vi "text_message_to_gemini_message.vi"(2 "error in (no error)":errorcluster, 3 "message":T2) -> (0 "error out":errorcluster, 1 "Content (JSON)":string)   [LabVIEW 2020, in "llm_gemini_chatmodels.lvclass"]
uses:
  llm_gemini_chatmodels.lvclass
  message_text/message.ctl
  message_text/message_text.lvclass
panel:
  out "Content":T1
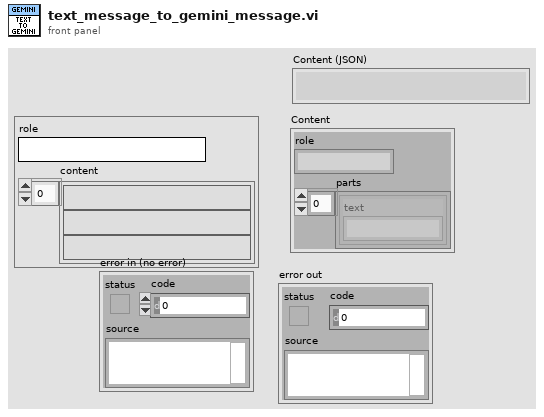
[diagram p1: front panel]
types:
  T1 = cluster{"role":string, "parts":cluster{"text":string}[]}
  T2 = typedef "message_text.lvclass/message.ctl" = cluster{"role":string, "content":string[]}
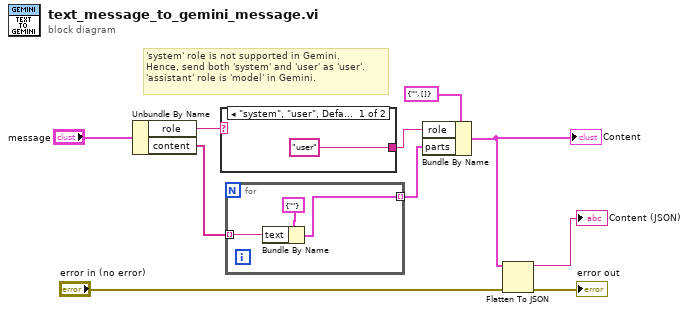
[diagram p0: block diagram]
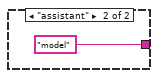
[diagram p2: hidden frame]
diagram:
  # "'system' role is not supported in Gemini.\nHence, send both 'system' and 'user' as 'user'.\n'assistant' role is 'model' in Gemini."
  n1 = Unbundle By Name("message") -> ("role"=w9:string, "content"=w6:string[])
  n2 = case shown="\"system\", \"user\", Default" w9 {
    tunnel: ["user" ("role") "model" ("role")] -> w8
    frame "system", "user", Default {
    }
    frame "assistant" {
    }
  }
  n3 = for {
    tunnel: w6 -> [w15] mode=indexing
    tunnel: [w13] -> w7 mode=indexing
    n4 = Bundle By Name(cluster=cluster{"text":string} {"text"=""} ("parts"), "text"=w15) -> (w13:cluster{"text":string})
  }
  n5 = Bundle By Name(cluster=T1 {"role"="", "parts"=[]} ("content"), "role"=w8, "parts"=w7) -> (w5:T1)
  "Content" <- w5
  n6 = Flatten To JSON(anything=w5, error in (no error)="error in (no error)") -> (JSON string=→"Content (JSON)":string, 11:→"error out":errorcluster)  [unwired: 1 in]
